vi "setSettings.vi"(8 "error in (no error)":errorcluster, 10 "SettingToApply":string, 11 "Boot in":refnum<class "Boot.lvclass">) -> (0 "error out":errorcluster, 3 "Boot out":refnum<class "Boot.lvclass">)   [LabVIEW 2016, in "Boot.lvclass"]
uses:
  Boot.lvclass
  Boot.lvclass/Boot.ctl
  Settings/Settings/Setting.lvclass/Setting.ctl
  Settings/Settings/Setting.lvclass
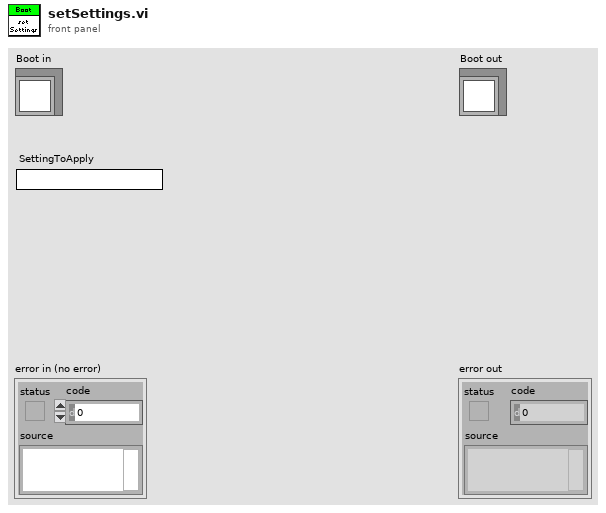
[diagram p1: front panel]
types:
  T1 = typedef "M1M3SupportSettings.lvlib/SettingAliases.ctl" = cluster{"Aliases":T2[]}
  T2 = typedef "M1M3SupportSettings.lvlib/SettingAlias.ctl" = cluster{"Alias":string, "Set":string, "Version":string}
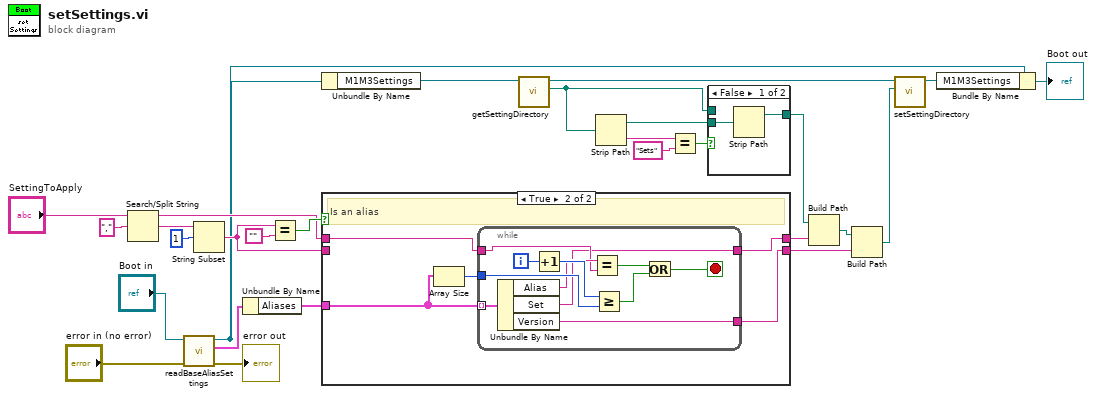
[diagram p0: block diagram]
diagram:
  n1 = Search/Split String(string="SettingToApply", search string/char (-)=",") -> (substring before match=w19:string, match + rest of string=w27:string)  [unwired: 1 in, 1 out]
  n2 = call "readBaseAliasSettings.vi"("error in (no error)"="error in (no error)", "Boot in"="Boot in") -> ("error out"=→"error out":errorcluster, "SettingAliases"=w21:T1, "Boot out"=w5:refnum<class "Boot.lvclass">)  [unwired: 7 in]
  n3 = String Subset(string=w27, offset (0)=1) -> (substring=w18:string)  [unwired: 1 in]
  n4 = Unbundle By Name(w21) -> ("Aliases"=w20:T2[])
  n5 = Equal?(x=w18, y="") -> (x = y?=w23:bool)
  n6 = Unbundle By Name(w5) -> ("M1M3Settings"=w17:refnum<class "Setting.lvclass">)
  n7 = case shown="True" w23 {
    tunnel: w20 -> [_ w35]
    tunnel: w19 -> [w30 w34]
    tunnel: w18 -> [w29 _]
    tunnel: [w30 w32] -> w9
    tunnel: [w29 w31] -> w7
    frame False {
      # "Isn't an alias"
    }
    frame True {
      # "Is an alias"
      n8 = Array Size(array=w35) -> (size(s)=w33:i32)
      n9 = while {
        tunnel: w35 -> [w46] mode=indexing
        tunnel: w34 -> [w39]
        tunnel: w33 -> [w43]
        tunnel: [w38] -> w32
        tunnel: [w37] -> w31
        i -> [w45]
        stop <- w41 stop-if-true
        n10 = Unbundle By Name(w46) -> ("Alias"=w40:string, "Set"=w38:string, "Version"=w37:string)
        n11 = Increment(x=w45) -> (x+1=w44:i32)
        n12 = Equal?(x=w40, y=w39) -> (x = y?=w36:bool)
        n13 = Greater Or Equal?(x=w44, y=w43) -> (x >= y?=w42:bool)
        n14 = Or(x=w36, y=w42) -> (x .or. y?=w41:bool)
      }
    }
  }
  n15 = call "getSettingDirectory.vi"("BaseSetting in"=w17) -> ("SettingDirectory"=w11:path, "BaseSetting out"=w16:refnum<class "Setting.lvclass">)  [unwired: 9 in]
  n16 = Strip Path(path=w11) -> (stripped path=w12:path, name=w15:string)
  n17 = Equal?(x=w15, y="Sets") -> (x = y?=w13:bool)
  n18 = case shown="False" w13 {
    tunnel: w12 -> [w48 _]
    tunnel: [w47 w49] -> w10
    tunnel: w11 -> [_ w49]
    frame False {
      n19 = Strip Path(path=w48) -> (stripped path=w47:path)  [unwired: 1 out]
    }
    frame True {
    }
  }
  n20 = Build Path(base path=w10, name or relative path=w9) -> (appended path=w8:path)
  n21 = Build Path(base path=w8, name or relative path=w7) -> (appended path=w6:path)
  n22 = call "setSettingDirectory.vi"("SettingDirectory"=w6, "BaseSetting in"=w16) -> ("BaseSetting out"=w4:refnum<class "Setting.lvclass">)  [unwired: 9 in]
  n23 = Bundle By Name(cluster=w5, "M1M3Settings"=w4) -> (→"Boot out":refnum<class "Boot.lvclass">)
